vi "Unflatten to PDU.vi"(8 "error in":errorcluster, 10 "modbus data unit data":u8[](array[numeric])) -> (0 "error out":errorcluster, 3 "modbus data unit out":refnum<class "Modbus Data Unit.lvclass">)   [LabVIEW 2012, in "Modbus Data Unit.lvclass"]
uses:
  Modbus Data Unit.lvclass
  Modbus Data Unit.lvclass/Modbus Data Unit.ctl
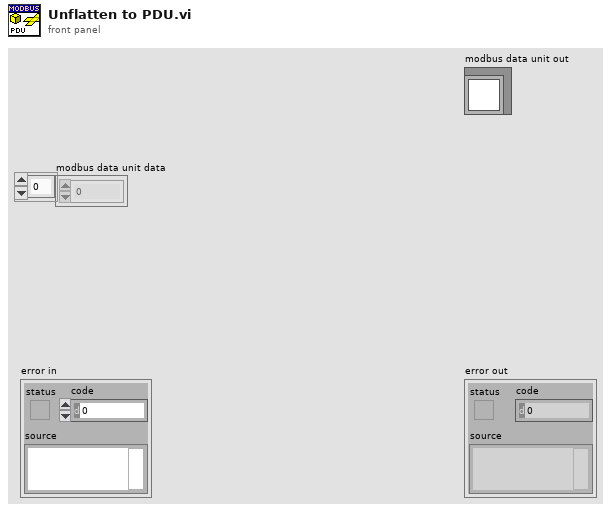
[diagram p1: front panel]
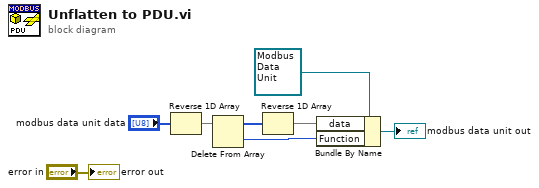
[diagram p0: block diagram]
diagram:
  n1 = Reverse 1D Array(array="modbus data unit data") -> (reversed array=w3:u8[])
  n2 = Delete From Array(array=w3) -> (deleted portion=w5:u8, array with subset deleted=w1:u8[])  [unwired: 2 in]
  n3 = Reverse 1D Array(array=w1) -> (reversed array=w2:u8[])
  n4 = Bundle By Name(cluster=refnum<class "Modbus Data Unit.lvclass"> refnum ("modbus data unit"), "data"=w2, "Function"=w5) -> (→"modbus data unit out":refnum<class "Modbus Data Unit.lvclass">)
  "error out" <- "error in"
